vi "ImageColorU64ToArray.vi"(8 "error in":errorcluster, 10 "Optional Rectangle":T1, 11 "Image Reference In":T2) -> (0 "error out":errorcluster, 2 "Pixel":u64[][](array[numeric]), 3 "Image Reference Out":T2)   [LabVIEW 2024, in "OpenLvVision_Image.lvlib" / "DataAccess.lvlib"]
doc: "Copies the pixel into an 2D array without an border."
uses:
  DataAccess.lvlib
  Management/TypeDef/Image.ctl
  TypeDef/RectangleI32.ctl
  TypeDef/StepSizes.ctl
  Management/Management.lvlib
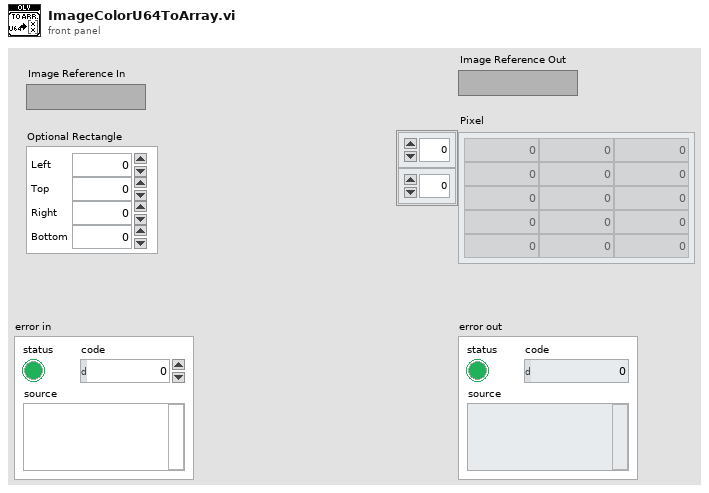
[diagram p1: front panel]
types:
  T1 = typedef "OpenLvVision_Image.lvlib/DataAccess.lvlib/RectangleI32.ctl" = cluster{"Left":i32, "Top":i32, "Right":i32, "Bottom":i32}
  T2 = typedef "OpenLvVision_Image.lvlib/Management.lvlib/Image.ctl" = refnum<image>
  T3 = typedef "OpenLvVision_Image.lvlib/DataAccess.lvlib/StepSizes.ctl" = cluster{"X Step Size":u32, "Y Step Size":u32}
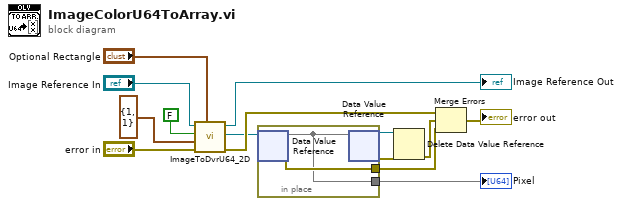
[diagram p0: block diagram]
diagram:
  n1 = call "ImageToDvrU64_2D.vi"("Optional Rectangle"="Optional Rectangle", "error in"="error in", "Step Sizes"=T3 {"X Step Size"=1, "Y Step Size"=1}, "Include Border"=FALSE, "Image Reference In"="Image Reference In") -> ("error out"=w7:errorcluster, "EDVR 2D U64"=w6:refnum<data-value>, "Image Reference Out"=→"Image Reference Out":T2)  [unwired: 3 in, 1 out]
  n2 = in-place {
    in-place-border: [w15] -> w8
    in-place-border: [w16] -> w5
    n3 = in-place-dvr #1(w6) -> (w15:u64[][], w16:errorcluster)
    n4 = in-place-dvr #1(w15) -> (w2:refnum<data-value>, w3:errorcluster)
  }
  "Pixel" <- w8
  n5 = Delete Data Value Reference(data value reference=w2, error in=w3) -> (error out=w1:errorcluster)  [unwired: 1 out]
  n6 = Merge Errors(w7, w1, w5) -> (→"error out":errorcluster)
